vi "pr5.vi"() -> ()   [LabVIEW 2014]
uses:
  <vilib>/measure/NI_MABase.lvlib
  <vilib>/sound2/lvsound2.llb/Sampling Mode.ctl
  <vilib>/sound2/lvsound2.llb/Sound Data Format.ctl
  Ctls/_ADC_ Supply Variables.ctl
  Ctls/_ADC_ Internal Variables.ctl
  <vilib>/sound2/lvsound2.llb/Sound Output Write (DBL).vi
  <vilib>/Analysis/3filter.llb/Filter Passband Type.ctl
  <vilib>/Analysis/NI_AALBase.lvlib
panel:
  in  "Signal Generation":T1={"Wave Type"=enum."Sine", "Wave Freq"=10.0, "Wave Amp"=1.0, "Wave Fs"=44100.0} {"Wave Fs" min=1000.0 max=1000000.0 step=1.0; "Wave Amp" min=0.0 max=12.0 step=0.0001 format="%.4f"; "Wave Freq" min=10.0 max=22000.0 step=1.0 format="%_4f"}
  out "Tab Control":enum32{"Page 1", "Page 2"}(tab)
  in  "Wave Freq 2":dbl=10.0 caption="2: Signal Frequency [Hz]" min=10.0 max=22000.0 step=1.0 format="%_4f"
  in  "Wave Amp 2":dbl=1.0 caption="2: Signal Amplitude [V]" min=0.0 max=12.0 step=0.0001 format="%.4f"
  in  "Noise Control":bool
  out "Signal Preview":waveform(dbl)[](graph)
  in  "Media Stop Button":bool
  in  "Import File":bool
  in  "Play Button":bool
  in  "Filter Creation":T3={"filter type"=enum."Lowpass", "high cutoff freq: fh"=0.45000000000000007, "low cutoff freq: fl"=0.12500000000000006, "order"=2} {"low cutoff freq: fl" min=0.0 max=22049.0 format="%0.4f"; "high cutoff freq: fh" min=500.0 max=22049.0 format="%0.2f"}
  in  "ADC Configuration":T4={"ADC V-"=-3.3, "ADC V+"=3.3, "ADC Res"=32, "ADC Fs"=44100.0} {"ADC Fs" min=10.0 max=1000000.0 step=1.0; "ADC Res" min=1 max=32 step=1; "ADC V+" min=-12.0 max=12.0 step=1e-05 format="%.4f"; "ADC V-" min=-12.0 max=12.0 step=1e-05 format="%.4f"}
  in  "Waveform Tab":T5(tab)
  out "Signal Overview":waveform(dbl)[](graph)
  out "FFT Overview":cluster{"f0":dbl, "df":dbl, "magnitude":dbl[]}[](graph)
  out "Filter Overview":cluster{"f0":dbl, "df":dbl, "magnitude":dbl[]}(graph)
  in  "Stop Button":bool
  # "PSI3214"
  # "Laboratório de Instrumentação Elétrica"
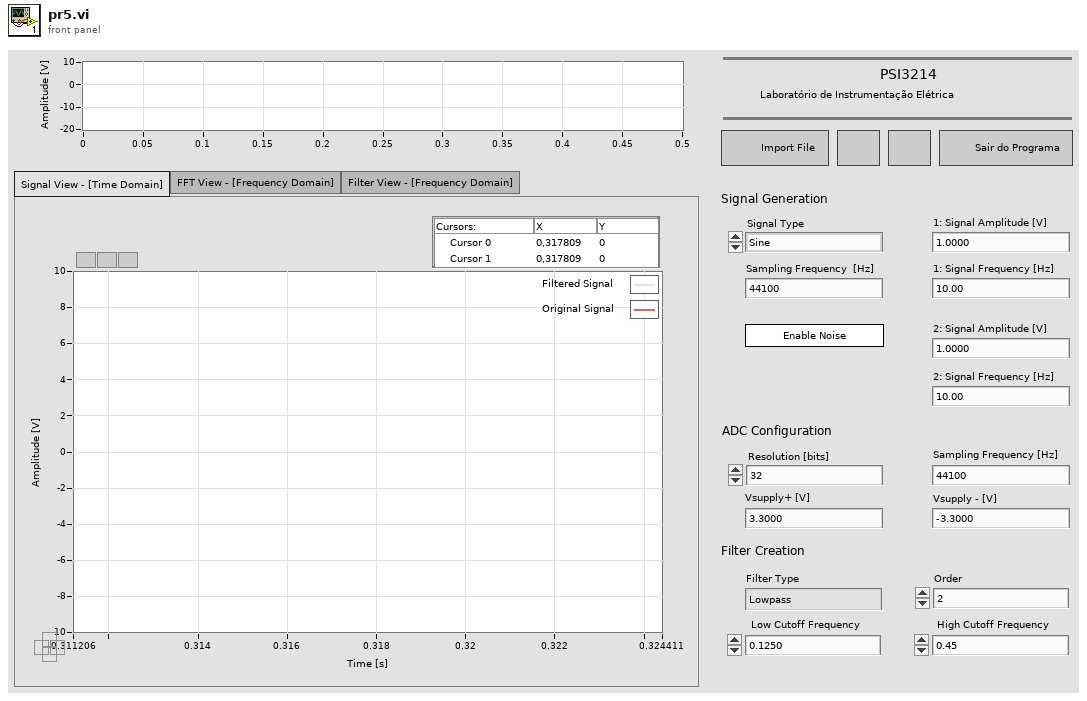
[diagram p1: front panel]
types:
  T1 = cluster{"Wave Type":enum16{"Sine", "Square", "Ramp", "White Noise", "Bimodal Sine"}, "Wave Freq":dbl, "Wave Amp":dbl, "Wave Fs":dbl}
  T2 = typedef "NI_AALBase.lvlib/Filter Passband Type.ctl" = enum32{"Lowpass", "Highpass", "Bandpass", "Bandstop"}
  T3 = cluster{"filter type":T2, "high cutoff freq: fh":dbl, "low cutoff freq: fl":dbl, "order":i32}
  T4 = cluster{"ADC V-":dbl, "ADC V+":dbl, "ADC Res":u8, "ADC Fs":dbl}
  T5 = enum32{"Signal View - [Time Domain]", "FFT View - [Frequency Domain]", "Filter View - [Frequency Domain]"}
  T6 = typedef "Sound Data Format.ctl" = cluster{"sample rate (S/s)":dbl, "number of channels":i32, "bits per sample":i32}
  T7 = typedef "Sampling Mode.ctl" = i32
  T8 = typedef "Sound Output Task ID.ctl" = u32
  T9 = typedef "_ADC_ Internal Variables.ctl" = cluster{"ADC Resolution":enum16{"0", "1", "2", "3", "4", "5", "6", "7", "8", "9", "10", "11", "12", "13", "14", "15", "16", "17", "18", "19", "20", "21", "22", "23", "24", "25", "26", "27", "28", "29", "30", "31", "32"}, "ADC Gain Error":dbl, "ADC Offset Error":dbl, "ADC Sampling Frequency Jitter":dbl, "ADC Sampling Frequency":dbl}
  T10 = typedef "_ADC_ Supply Variables.ctl" = cluster{"ADC Supply Ripple Frequency":dbl, "Gen Wave Sampling Frequency":dbl, "ADC Neg Supply Ripple Amplitude":dbl, "ADC Neg Supply Offset":dbl, "ADC Pos Supply Ripple Amplitude":dbl, "ADC Pos Supply Offset":dbl, "ADC Supply Diff Noise Amplitude":dbl}
  T11 = typedef "LVPoint32TypeDef.ctl" = cluster{"Horizontal":i32, "Vertical":i32}
  T12 = enum16{"Sine", "Square", "Ramp", "White Noise", "Bimodal Sine"}
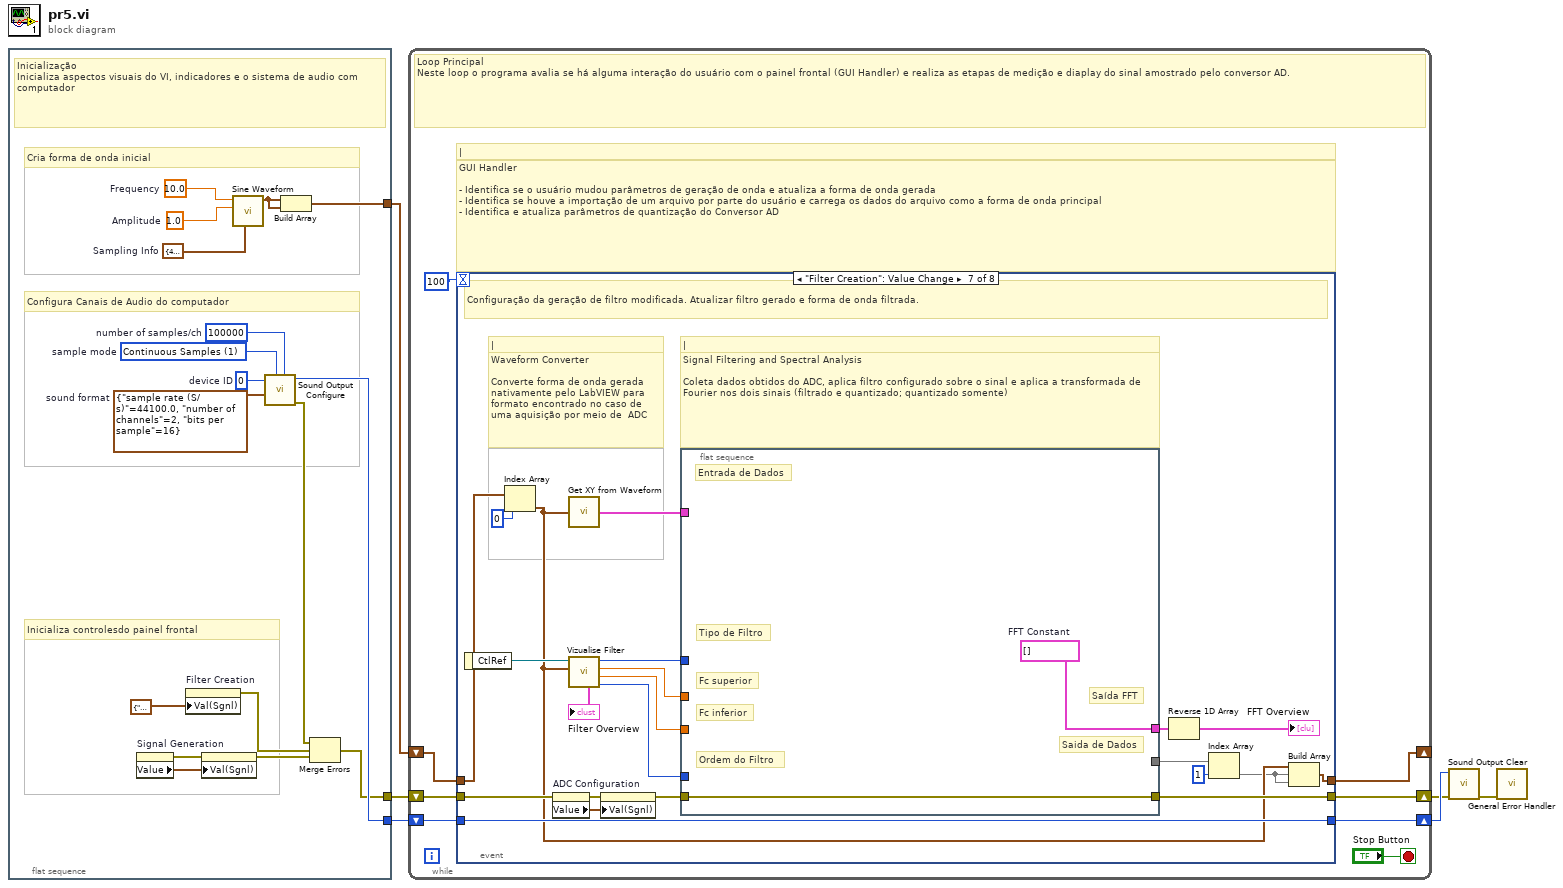
[diagram p0: block diagram]
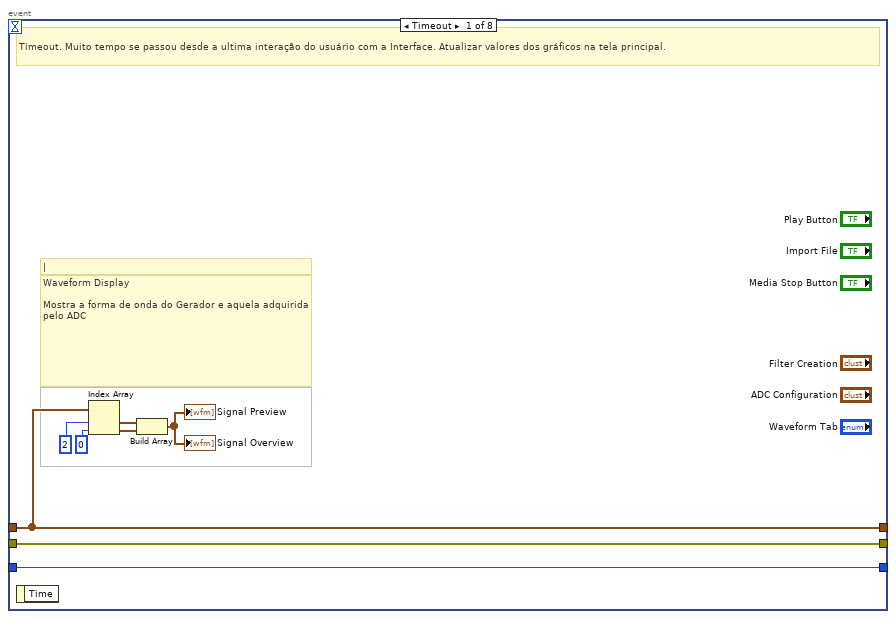
[diagram p2: hidden frame]
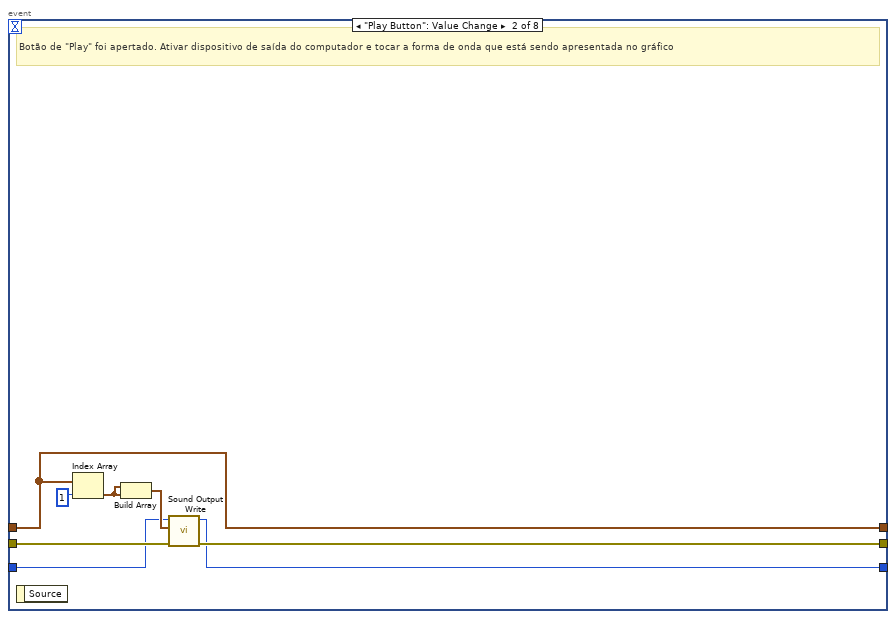
[diagram p3: hidden frame]
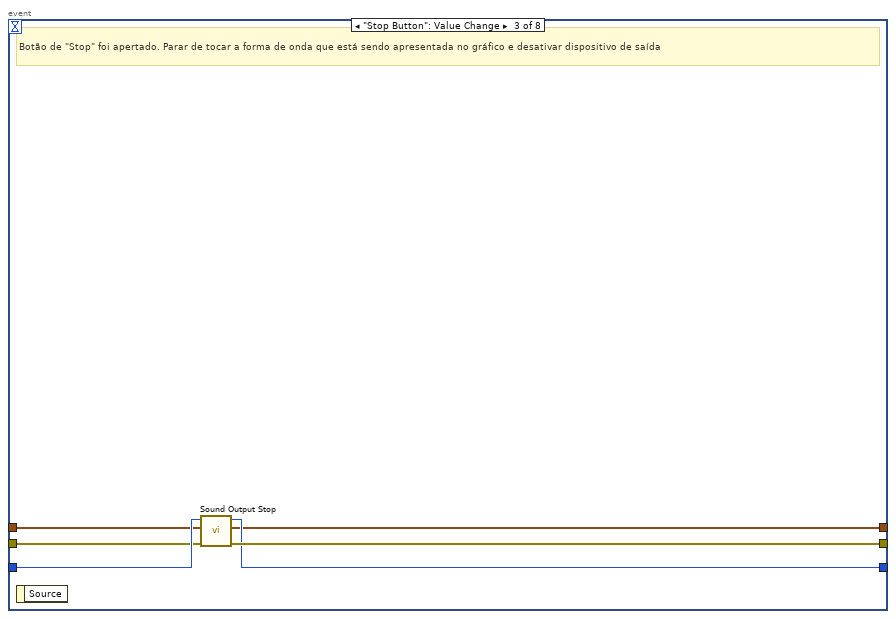
[diagram p4: hidden frame]
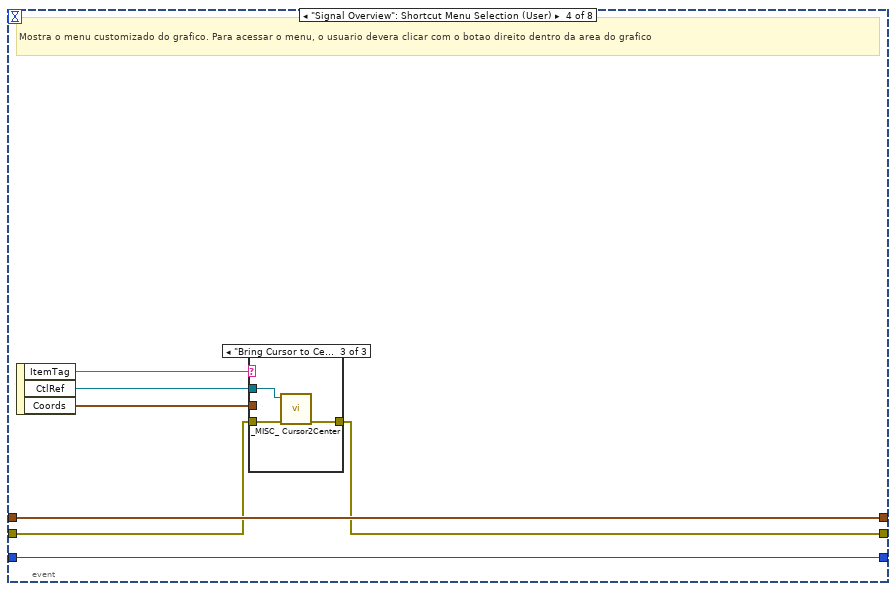
[diagram p5: hidden frame]
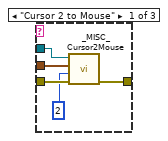
[diagram p6: hidden frame]
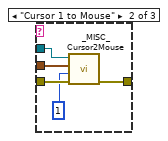
[diagram p7: hidden frame]
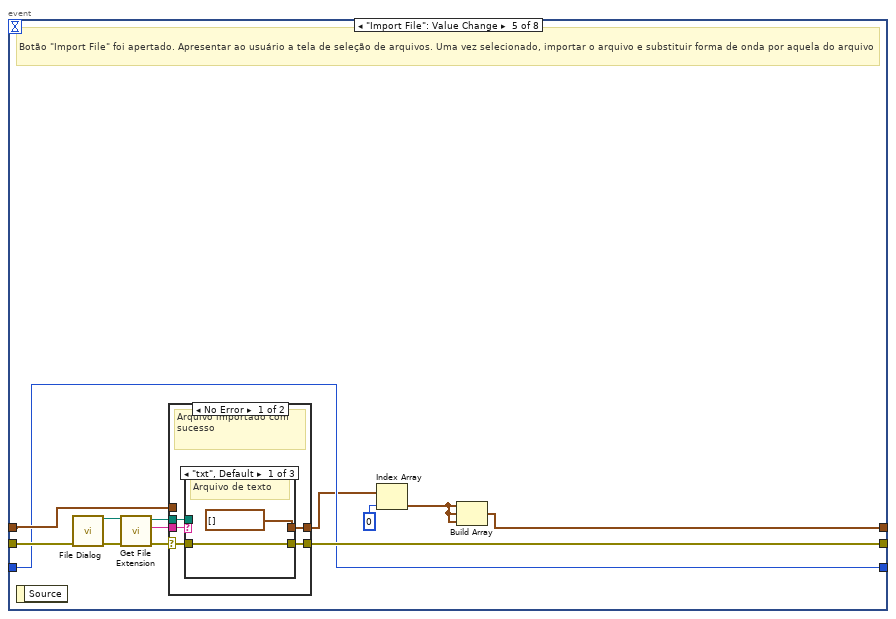
[diagram p8: hidden frame]
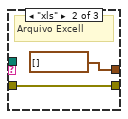
[diagram p9: hidden frame]
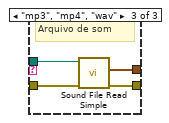
[diagram p10: hidden frame]
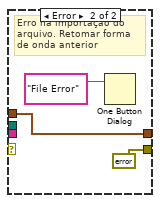
[diagram p11: hidden frame]
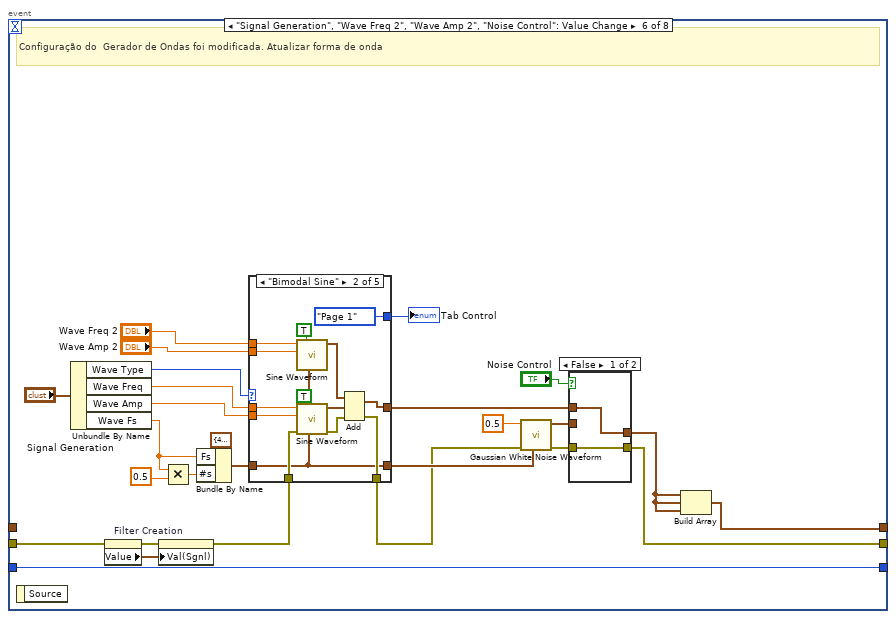
[diagram p12: hidden frame]
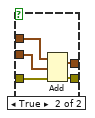
[diagram p13: hidden frame]
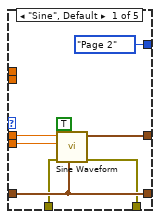
[diagram p14: hidden frame]
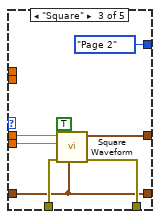
[diagram p15: hidden frame]
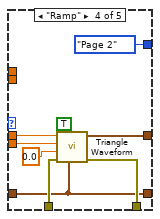
[diagram p16: hidden frame]
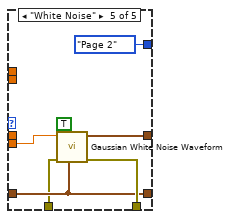
[diagram p17: hidden frame]
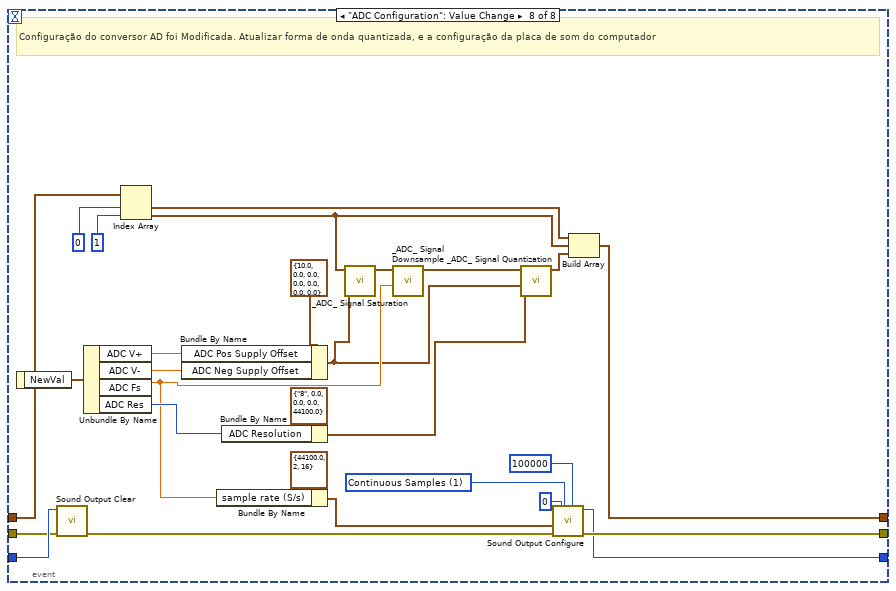
[diagram p18: hidden frame]
diagram:
  n1 = flat-sequence {
    tunnel: [w19] -> w5
    tunnel: [w12] -> w4
    tunnel: [w14] -> w1
    frame #0 {
      w15 = T6 {"sample rate (S/s)"=44100.0, "number of channels"=2, "bits per sample"=16}  # sound format
      w16 = 100000  # number of samples/ch
      w17 = T7 1 items=["Finite Samples", "Continuous Samples"]  # sample mode
      w18 = u32 0  # device ID
      w20 = cluster{"Fs":dbl, "#s":dbl} {"Fs"=44100.0, "#s"=44100.0}  # Sampling Info
      w22 = 10.0  # Frequency
      w23 = 1.0  # Amplitude
      # "Inicializa controlesdo painel frontal"
      # "Configura Canais de Audio do computador"
      # "Cria forma de onda inicial"
      # "Inicialização\nInicializa aspectos visuais do VI, indicadores e o sistema de audio com computador"
      n2 = property on="Signal Generation" class="Clust (strict)"() -> (error out=w11:errorcluster, "Value"=w10:T1)  [unwired: 2 in, 1 out]
      n3 = property on="Filter Creation" class="Clust (strict)"("Val(Sgnl)"=T3 {"filter type"=enum."Lowpass", "high cutoff freq: fh"=0.45000000000000007, "low cutoff freq: fl"=5000.0, "order"=2} ("Filter Creation")) -> (error out=w8:errorcluster)  [unwired: 2 in, 1 out]
      n4 = property on="Signal Generation" class="Clust (strict)"(error in=w11, "Val(Sgnl)"=w10) -> (error out=w9:errorcluster)  [unwired: 1 in, 1 out]
      n5 = call <vilib>:"Sine Waveform.vi"("sampling info"=w20, "amplitude"=w23, "frequency"=w22) -> ("signal out"=w21:waveform(dbl))  [unwired: 7 in, 1 out]
      n6 = call <vilib>:"Sound Output Configure.vi"("number of samples/ch"=w16, "sample mode"=w17, "sound format"=w15, "device ID"=w18) -> ("error out"=w13:errorcluster, "task ID"=w14:T8)  [unwired: 6 in]
      n7 = Build Array(w21, w21) -> (w19:waveform(dbl)[])
      n8 = Merge Errors(w13, w8, w9) -> (w12:errorcluster)
    }
  }
  n9 = while {
    shift-right: [w25] -> _
    shift-left: w5 -> [w30]
    shift-right: [w27] -> w6
    shift-left: w1 -> [w31]
    shift-right: [w28] -> w3
    shift-left: w4 -> [w29]
    stop <- "Stop Button" stop-if-true
    # "GUI Handler\n\n- Identifica se o usuário mudou parâmetros de geração de onda e atualiza a forma de onda gerada\n- Identifica se houve a importação de um arquivo por parte do usuário e carrega os dados do arquivo como a forma de onda principal\n- Identifica e atualiza parâmetros de quantização do Conversor AD"
    # "|"
    # "Loop Principal\nNeste loop o programa avalia se há alguma interação do usuário com o painel frontal (GUI Handler) e realiza as etapas de medição e diaplay do sinal amostrado pelo conversor AD."
    n10 = event shown="[6] \"Filter Creation\": Value Change" {
      selector: _ -> [_ _ _ _ _ _ _ _]
      dyn-events: _ -> [_ _ _ _ _ _ _ _]
      timeout: 100 -> [_ _ _ _ _ _ _ _]
      tunnel: w31 -> [w39 w42 w52 w59 w77 w128 w203 w222]
      tunnel: w30 -> [w33 w40 w48 w58 w80 _ w197 w223]
      tunnel: w29 -> [w38 w44 w51 w57 w79 w104 w188 w221]
      tunnel: [w38 w43 w50 w56 w78 w107 w198 w220] -> w28
      tunnel: [w39 w41 w49 w59 w77 w128 w203 w218] -> w27
      tunnel: [w33 w40 w48 w58 w73 w119 w185 w219] -> w25
      event Timeout {
        # "|"
        # "Waveform Display\n\nMostra a forma de onda do Gerador e aquela adquirida pelo ADC"
        # "Timeout. Muito tempo se passou desde a ultima interação do usuário com a Interface. Atualizar valores dos gráficos na tela principal."
        n11 = event-data() -> ()  [unwired: 1 in, 1 out]
        n12 = Index Array(array=w33, index #1=2 ("index"), index #2=0 ("index")) -> (element #1=w35:waveform(dbl), element #2=w34:waveform(dbl))
        n13 = Build Array(w35, w34) -> (→"Signal Preview" →"Signal Overview":waveform(dbl)[])
      }
      event "Play Button": Value Change {
        # "Botão de \"Play\" foi apertado. Ativar dispositivo de saída do computador e tocar a forma de onda que está sendo apresentada no gráfico"
        n14 = event-data() -> ()  [unwired: 1 in, 1 out]
        n15 = Index Array(array=w40, index=1) -> (element=w46:waveform(dbl))
        n16 = Build Array(w46, w46) -> (w45:waveform(dbl)[])
        n17 = call-poly <vilib>:"Sound Output Write.vi"("error in (no error)"=w44, "data"=w45, "task ID"=w42) -> ("error out"=w43:errorcluster, "task ID out"=w41:T8)  [unwired: 7 in]
      }
      event "Stop Button": Value Change {
        # "Botão de \"Stop\" foi apertado. Parar de tocar a forma de onda que está sendo apresentada no gráfico e desativar dispositivo de saída"
        n18 = event-data() -> ()  [unwired: 1 in, 1 out]
        n19 = call <vilib>:"Sound Output Stop.vi"("error in (no error)"=w51, "task ID"=w52) -> ("error out"=w50:errorcluster, "task ID out"=w49:T8)  [unwired: 8 in]
      }
      event "Signal Overview": Shortcut Menu Selection (User) {
        # "Mostra o menu customizado do grafico. Para acessar o menu, o usuario devera clicar com o botao direito dentro da area do grafico"
        n20 = event-data() -> ("ItemTag"=w55:string, "CtlRef"=w54:refnum<vi>, "Coords"=w53:T11)  [unwired: 1 in]
        n21 = case shown="\"Bring Cursor to Center\", Default" w55 {
          tunnel: w57 -> [w64 w69 w72]
          tunnel: [w63 w65 w71] -> w56
          tunnel: w54 -> [w60 w66 w70]
          tunnel: w53 -> [w61 w67 _]
          frame "Cursor 2 to Mouse" {
            n22 = call "_MISC_ Cursor2Mouse.vi"("Error In"=w64, "Cursor Index"=2, "Coords"=w61, "WaveformGraph Ref"=w60) -> ("Error out"=w63:errorcluster)  [unwired: 6 in, 1 out]
          }
          frame "Cursor 1 to Mouse" {
            n23 = call "_MISC_ Cursor2Mouse.vi"("Error In"=w69, "Cursor Index"=1, "Coords"=w67, "WaveformGraph Ref"=w66) -> ("Error out"=w65:errorcluster)  [unwired: 6 in, 1 out]
          }
          frame "Bring Cursor to Center", Default {
            n24 = call "_MISC_ Cursor2Center.vi"("Error In"=w72, "WaveformGraph Ref"=w70) -> ("Error Out"=w71:errorcluster)  [unwired: 8 in, 1 out]
          }
        }
      }
      event "Import File": Value Change {
        # "Botão \"Import File\" foi apertado. Apresentar ao usuário a tela de seleção de arquivos. Uma vez selecionado, importar o arquivo e substituir forma de onda por aquela do arquivo"
        n25 = event-data() -> ()  [unwired: 1 in, 1 out]
        n26 = call "File Dialog"("error in"=w79) -> ("selected path"=w82:path, "error out"=w85:errorcluster)  [unwired: 11 in, 2 out]
        n27 = call <vilib>:"Get File Extension.vi"("error in (no error)"=w85, "file"=w82) -> ("error out"=w84:errorcluster, "lowercase file extension"=w83:string, "dup file"=w81:path)  [unwired: 6 in, 1 out]
        n28 = case shown="No Error" w84 {
          selector: w84 -> [w88 _]
          tunnel: [w87 errorcluster {"status"=FALSE, "code"=0, "source"=""} ("error constant")] -> w78
          tunnel: w83 -> [w90 _]
          tunnel: w81 -> [w89 _]
          tunnel: [w86 w99] -> w74
          tunnel: w80 -> [_ w99]
          frame No Error {
            # "Arquivo importado com sucesso"
            n29 = case shown="\"txt\", Default" w90 {
              tunnel: w89 -> [_ _ w98]
              tunnel: w88 -> [w92 w94 w97]
              tunnel: [w92 w94 w96] -> w87
              tunnel: [waveform(dbl)[] [] ("data") waveform(dbl)[] [] ("data") w95] -> w86
              frame "txt", Default {
                # "Arquivo de texto"
              }
              frame "xls" {
                # "Arquivo Excell"
              }
              frame "mp3", "mp4", "wav" {
                # "Arquivo de som"
                n30 = call <vilib>:"Sound File Read Simple.vi"("error in (no error)"=w97, "path"=w98) -> ("error out"=w96:errorcluster, "data"=w95:waveform(dbl)[])  [unwired: 6 in, 2 out]
              }
            }
          }
          frame Error {
            # "Erro na importação do arquivo. Retomar forma de onda anterior"
            n31 = One Button Dialog(message="File Error") -> ()  [unwired: 1 in, 1 out]
          }
        }
        n32 = Index Array(array=w74, index=0) -> (element=w75:waveform(dbl))
        n33 = Build Array(w75, w75, w75) -> (w73:waveform(dbl)[])
      }
      event "Signal Generation", "Wave Freq 2", "Wave Amp 2", "Noise Control": Value Change {
        # "Configuração do  Gerador de Ondas foi modificada. Atualizar forma de onda"
        n34 = event-data() -> ()  [unwired: 1 in, 1 out]
        n35 = Unbundle By Name("Signal Generation") -> ("Wave Type"=w123:T12, "Wave Freq"=w122:dbl, "Wave Amp"=w121:dbl, "Wave Fs"=w120:dbl)
        n36 = property on="Filter Creation" class="Clust (strict)"(error in=w104) -> (error out=w105:errorcluster, "Value"=w106:T3)  [unwired: 1 in, 1 out]
        n37 = property on="Filter Creation" class="Clust (strict)"(error in=w105, "Val(Sgnl)"=w106) -> (error out=w103:errorcluster)  [unwired: 1 in, 1 out]
        n38 = Multiply(x=w120, y=0.5) -> (x*y=w125:dbl)
        n39 = Bundle By Name(cluster=cluster{"Fs":dbl, "#s":dbl} {"Fs"=44100.0, "#s"=4410.0} ("Spl Info"), "Fs"=w120, "#s"=w125) -> (w126:cluster{"Fs":dbl, "#s":dbl})
        n40 = case shown="\"Bimodal Sine\"" w123 {
          tunnel: w126 -> [w143 w144 w160 w170 w180]
          tunnel: w122 -> [w142 w157 w162 w172 _]
          tunnel: w121 -> [w141 w156 w161 w171 w177]
          tunnel: w103 -> [w140 w155 w165 w174 w178]
          tunnel: [w139 w146 w164 w173 w181] -> w110
          tunnel: [w138 w145 w163 w168 w179] -> w111
          tunnel: "Wave Amp 2" -> [_ w152 _ _ _]
          tunnel: "Wave Freq 2" -> [_ w151 _ _ _]
          tunnel: [enum32{"Page 1", "Page 2"}."Page 2" ("Tab Control") enum32{"Page 1", "Page 2"}."Page 1" ("Tab Control") enum32{"Page 1", "Page 2"}."Page 2" ("Tab Control") enum32{"Page 1", "Page 2"}."Page 2" ("Tab Control") enum32{"Page 1", "Page 2"}."Page 2" ("Tab Control")] -> w115
          tunnel: [w143 w144 w160 w170 w180] -> w114
          frame "Sine", Default {
            n41 = call <vilib>:"Sine Waveform.vi"("sampling info"=w143, "reset signal"=TRUE, "error in (no error)"=w140, "amplitude"=w141, "frequency"=w142) -> ("error out"=w139:errorcluster, "signal out"=w138:waveform(dbl))  [unwired: 5 in]
          }
          frame "Bimodal Sine" {
            n42 = call <vilib>:"Sine Waveform.vi"("sampling info"=w144, "reset signal"=TRUE, "amplitude"=w152, "frequency"=w151) -> ("signal out"=w148:waveform(dbl))  [unwired: 6 in, 1 out]
            n43 = call <vilib>:"Sine Waveform.vi"("sampling info"=w144, "reset signal"=TRUE, "error in (no error)"=w155, "amplitude"=w156, "frequency"=w157) -> ("error out"=w147:errorcluster, "signal out"=w149:waveform(dbl))  [unwired: 5 in]
            n44 = Add(1:w149, 2:w148, 4:w147) -> (0:w145:waveform(dbl), 3:w146:errorcluster)
          }
          frame "Square" {
            n45 = call <vilib>:"Square Waveform.vi"("sampling info"=w160, "reset signal"=TRUE, "error in (no error)"=w165, "amplitude"=w161, "frequency"=w162) -> ("error out"=w164:errorcluster, "signal out"=w163:waveform(dbl))  [unwired: 5 in]
          }
          frame "Ramp" {
            n46 = call <vilib>:"Triangle Waveform.vi"("sampling info"=w170, "reset signal"=TRUE, "error in (no error)"=w174, "phase"=0.0, "amplitude"=w171, "frequency"=w172) -> ("error out"=w173:errorcluster, "signal out"=w168:waveform(dbl))  [unwired: 4 in]
          }
          frame "White Noise" {
            n47 = call <vilib>:"Gaussian White Noise Waveform.vi"("sampling info"=w180, "reset signal"=TRUE, "error in (no error)"=w178, "standard deviation"=w177) -> ("error out"=w181:errorcluster, "signal out"=w179:waveform(dbl))  [unwired: 6 in]
          }
        }
        "Tab Control" <- w115
        n48 = call <vilib>:"Gaussian White Noise Waveform.vi"("sampling info"=w114, "error in (no error)"=w110, "standard deviation"=0.5) -> ("error out"=w109:errorcluster, "signal out"=w108:waveform(dbl))  [unwired: 7 in]
        n49 = case shown="False" "Noise Control" {
          tunnel: w111 -> [w129 w133]
          tunnel: w109 -> [w130 w134]
          tunnel: w108 -> [_ w135]
          tunnel: [w129 w132] -> w102
          tunnel: [w130 w131] -> w107
          frame False {
          }
          frame True {
            n50 = Add(1:w135, 2:w133, 4:w134) -> (0:w132:waveform(dbl), 3:w131:errorcluster)
          }
        }
        n51 = Build Array(w102, w102, w102) -> (w119:waveform(dbl)[])
      }
      event "Filter Creation": Value Change {
        # "Signal Filtering and Spectral Analysis\n\nColeta dados obtidos do ADC, aplica filtro configurado sobre o sinal e aplica a transformada de Fourier nos dois sinais (filtrado e quantizado; quantizado somente)"
        # "Waveform Converter\n\nConverte forma de onda gerada nativamente pelo LabVIEW para formato encontrado no caso de uma aquisição por meio de  ADC"
        # "|"
        # "|"
        # "Configuração da geração de filtro modificada. Atualizar filtro gerado e forma de onda filtrada."
        n52 = event-data() -> ("CtlRef"=w196:refnum<vi>)  [unwired: 1 in]
        n53 = Index Array(array=w197, index=0) -> (element=w184:waveform(dbl))
        n54 = property on="ADC Configuration" class="Clust (strict)"(error in=w188) -> (error out=w190:errorcluster, "Value"=w189:T4)  [unwired: 1 in, 1 out]
        n55 = call "Get XY from Waveform.vi"("Waveform In"=w184) -> ("XY Array Out"=w202:cluster{"Yo":dbl, "Xo":timestamp}[])
        n56 = call "Vizualise Filter.vi"("Reference Signal"=w184, "CtlRef"=w196) -> ("Order"=w192:i32, "Fc Low"=w193:dbl, "Fc High"=w194:dbl, "Type"=w195:T2, "Filter Magnitude"=→"Filter Overview":cluster{"f0":dbl, "df":dbl, "magnitude":dbl[]})  [unwired: 5 in]
        n57 = property on="ADC Configuration" class="Clust (strict)"(error in=w190, "Val(Sgnl)"=w189) -> (error out=w187:errorcluster)  [unwired: 1 in, 1 out]
        n58 = flat-sequence {
          tunnel: w202 -> [_]
          tunnel: [w204] -> w200
          tunnel: w187 -> [w205]
          tunnel: [w205] -> w198
          tunnel: w195 -> [_]
          tunnel: w194 -> [_]
          tunnel: w193 -> [_]
          tunnel: w192 -> [_]
          tunnel: [_] -> w183
          frame #0 {
            w204 = cluster{"f0":dbl, "df":dbl, "magnitude":dbl[]}[] []  # FFT Constant
            # "Saída FFT"
            # "Saida de Dados"
            # "Entrada de Dados"
            # "Ordem do Filtro"
            # "Fc inferior"
            # "Fc superior"
            # "Tipo de Filtro"
          }
        }
        n59 = Reverse 1D Array(array=w200) -> (reversed array=→"FFT Overview":cluster{"f0":dbl, "df":dbl, "magnitude":dbl[]}[])
        n60 = Index Array(array=w183, index=1) -> (element=w182)
        n61 = Build Array(w184, w182, w182) -> (w185:waveform(dbl)[])
      }
      event "ADC Configuration": Value Change {
        w228 = T7 1 items=["Finite Samples", "Continuous Samples"] ("sample mode")
        # "Configuração do conversor AD foi Modificada. Atualizar forma de onda quantizada, e a configuração da placa de som do computador"
        n62 = event-data() -> ("NewVal"=w224:T4)  [unwired: 1 in]
        n63 = call <vilib>:"Sound Output Clear.vi"("error in (no error)"=w221, "task ID"=w222) -> ("error out"=w206:errorcluster)  [unwired: 9 in]
        n64 = Unbundle By Name(w224) -> ("ADC V+"=w232:dbl, "ADC V-"=w231:dbl, "ADC Fs"=w215:dbl, "ADC Res"=w230:u8)
        n65 = Index Array(array=w223, index #1=0 ("index"), index #2=1 ("index")) -> (element #1=w210:waveform(dbl), element #2=w208:waveform(dbl))
        n66 = Bundle By Name(cluster=T10 {"ADC Supply Ripple Frequency"=10.0, "Gen Wave Sampling Frequency"=0.0, "ADC Neg Supply Ripple Amplitude"=0.0, "ADC Neg Supply Offset"=0.0, "ADC Pos Supply Ripple Amplitude"=0.0, "ADC Pos Supply Offset"=0.0, "ADC Supply Diff Noise Amplitude"=0.0} ("Cluster 2"), "ADC Pos Supply Offset"=w232, "ADC Neg Supply Offset"=w231) -> (w213:T10)
        n67 = Bundle By Name(cluster=T6 {"sample rate (S/s)"=44100.0, "number of channels"=2, "bits per sample"=16} ("sound format"), "sample rate (S/s)"=w215) -> (w225:T6)
        n68 = Bundle By Name(cluster=T9 {"ADC Resolution"=enum."8", "ADC Gain Error"=0.0, "ADC Offset Error"=0.0, "ADC Sampling Frequency Jitter"=0.0, "ADC Sampling Frequency"=44100.0} ("Cluster"), "ADC Resolution"=w230) -> (w214:T9)
        n69 = call "_ADC_ Signal Saturation.vi"("Supply Parameters"=w213, "Input Wave"=w208) -> ("Output Wave"=w217:waveform(dbl))  [unwired: 9 in]
        n70 = call "_ADC_ Signal Downsample.vi"("ADC Sampling Frequency"=w215, "Input Wave"=w217) -> ("Output Wave"=w216:waveform(dbl))  [unwired: 7 in]
        n71 = call "_ADC_ Signal Quantization.vi"("ADC Internal Parametes"=w214, "Supply Parameters"=w213, "Input Wave"=w216) -> ("Output Wave"=w207:waveform(dbl))  [unwired: 6 in]
        n72 = call <vilib>:"Sound Output Configure.vi"("number of samples/ch"=100000, "sample mode"=w228, "error in (no error)"=w206, "sound format"=w225, "device ID"=u32 0) -> ("error out"=w220:errorcluster, "task ID"=w218:T8)  [unwired: 5 in]
        n73 = Build Array(w210, w208, w207) -> (w219:waveform(dbl)[])
      }
    }
  }
  n74 = call <vilib>:"Sound Output Clear.vi"("error in (no error)"=w3, "task ID"=w6) -> ("error out"=w2:errorcluster)  [unwired: 9 in]
  n75 = call <vilib>:"General Error Handler.vi"("error in (no error)"=w2) -> ()  [unwired: 10 in, 5 out]
